vi "FGV_REWORK_DIAGNOSTICS_records_display.vi"(4 "front_panel_reference":refnum<vi>, 6 "SQL_listbox_reference":refnum<vi>, 7 "options":T2, 8 "error_in":errorcluster, 11 "input":variant) -> (0 "error_out":errorcluster, 1 "all_info":T1)   [LabVIEW 2019]
uses:
  FGV_REWORK_DIAGNOSTICS_records_display.ctl
  REWORK_DIAGNOSTICS_all_info.ctl
  ini/typedef/REWORK_all_config_info.ctl
  ini/typedef/REWORK_main_ini_file.ctl
  queues/typedef/REWORK_queue_refnums.ctl
  queues/typedef/REWORK_MAIN_queue_element.ctl
  MAIN/REWORK_MAIN_sequence_state.ctl
  queues/typedef/REWORK_SCANNER_queue_element.ctl
  SCANNER/REWORK_SCANNER_sequence_state.ctl
  _misc/PLC_connection_status.ctl
  connection_indicators/FGV_REWORK_connection_indicators.ctl
  _misc/AULocalize/SubVIs/Get Localized Phrase Compact Interface 1D.vi
  _misc/AULocalize/SubVIs/Get Localized Phrase Compact Interface 0D.vi
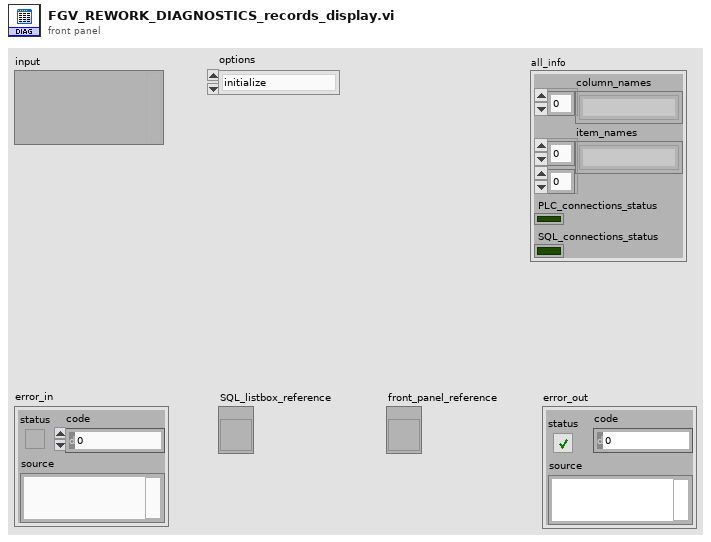
[diagram p1: front panel]
types:
  T1 = typedef "REWORK_DIAGNOSTICS_all_info.ctl" = cluster{"column_names":string[], "item_names":string[][], "PLC_connections_status":bool, "SQL_connections_status":bool}
  T2 = typedef "FGV_REWORK_DIAGNOSTICS_records_display.ctl" = enum16{"initialize", "set_PLC_IP", "set_PLC_Port", "set_PLC_connection_status", "set_SQL_connection_status", "get_all_info"}
  T3 = typedef "REWORK_all_config_info.ctl" = cluster{"main_ini_file":T4, "SQL Password":string, "queue_refnums":T5}
  T4 = typedef "REWORK_main_ini_file.ctl" = cluster{"SQL Driver":string, "SQL Server":string, "SQL Database":string, "SQL UID":string, "User table":string, "default language":string, "SCANNER COM port":u16, "SCANNER Baud rate":u32, "SCANNER Data bits":u16, "SCANNER Pairity":enum16{"None", "Odd", "Even", "Mark", "Space"}, "SCANNER Stop bits":u16, "SCANNER Flow control":u16, "SCANNER Termination char":u8, "ST 140 name":string, "ST 140 listener IP":string, "ST 140 listener port":u16, "logout timeout [ms]":i32}
  T5 = typedef "REWORK_queue_refnums.ctl" = cluster{"MAIN_queue":refnum<queue>, "SCANNER_queue":refnum<queue>, "SCANNER_data":refnum<queue>}
  T6 = typedef "FGV_REWORK_connection_indicators.ctl" = enum16{"initialize", "SQL_conn_ind_update", "PLC_conn_ind_update"}
  T7 = typedef "PLC_connection_status.ctl" = enum16{"Connected", "Waiting", "Error", "-"}
  T8 = cluster{"index (row)":i32, "disabled index (col)":i32}
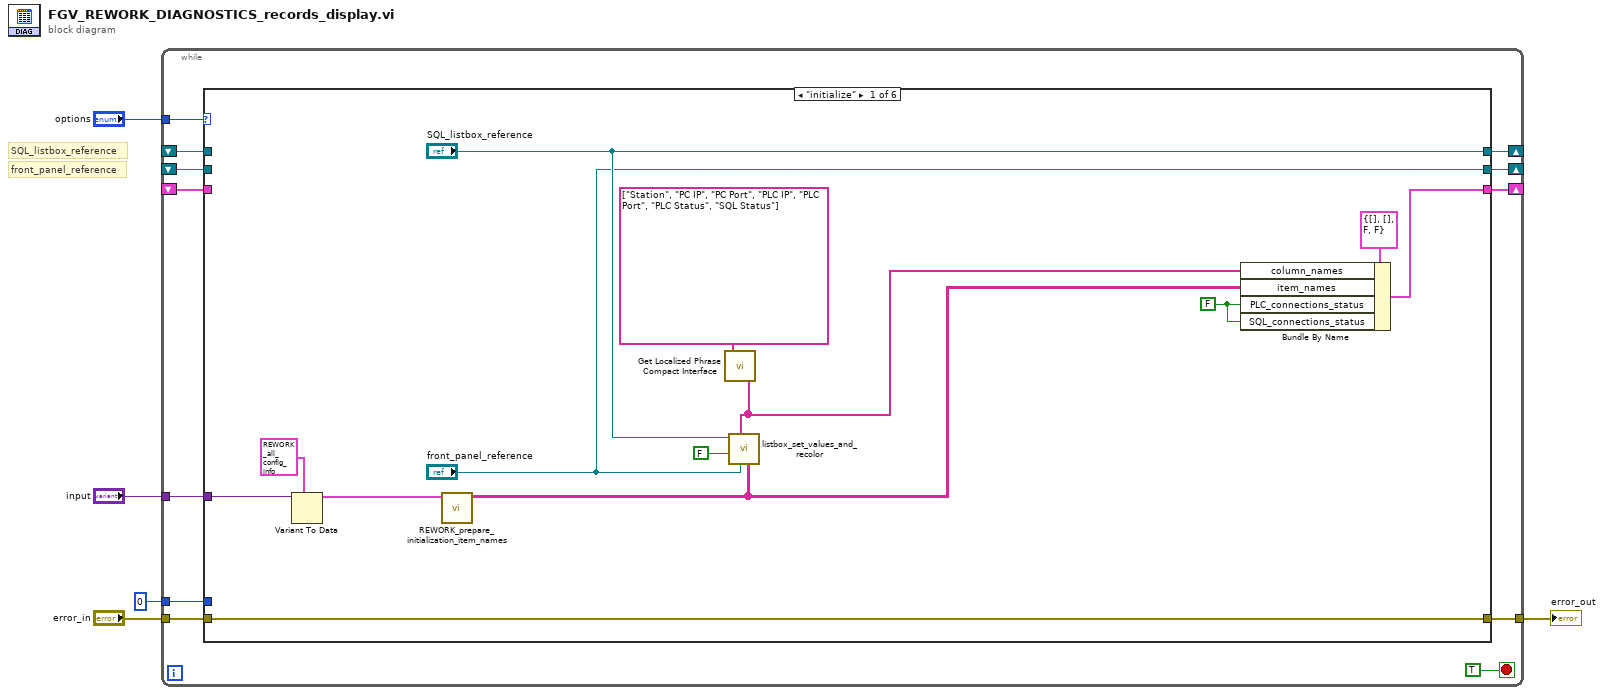
[diagram p0: block diagram]
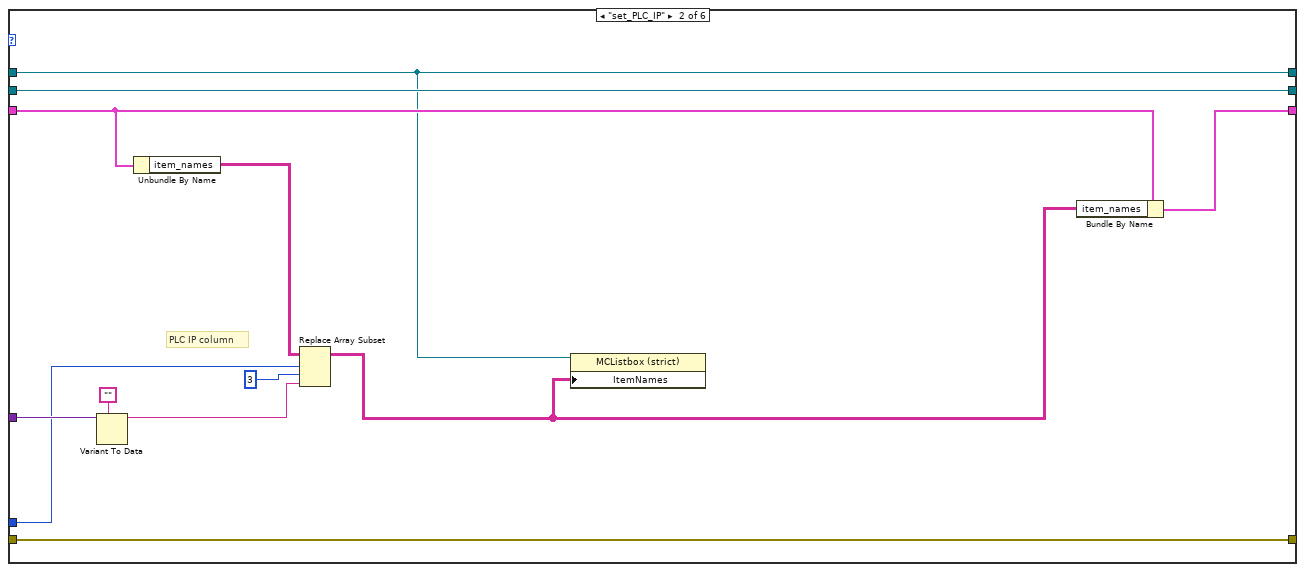
[diagram p2: hidden frame]
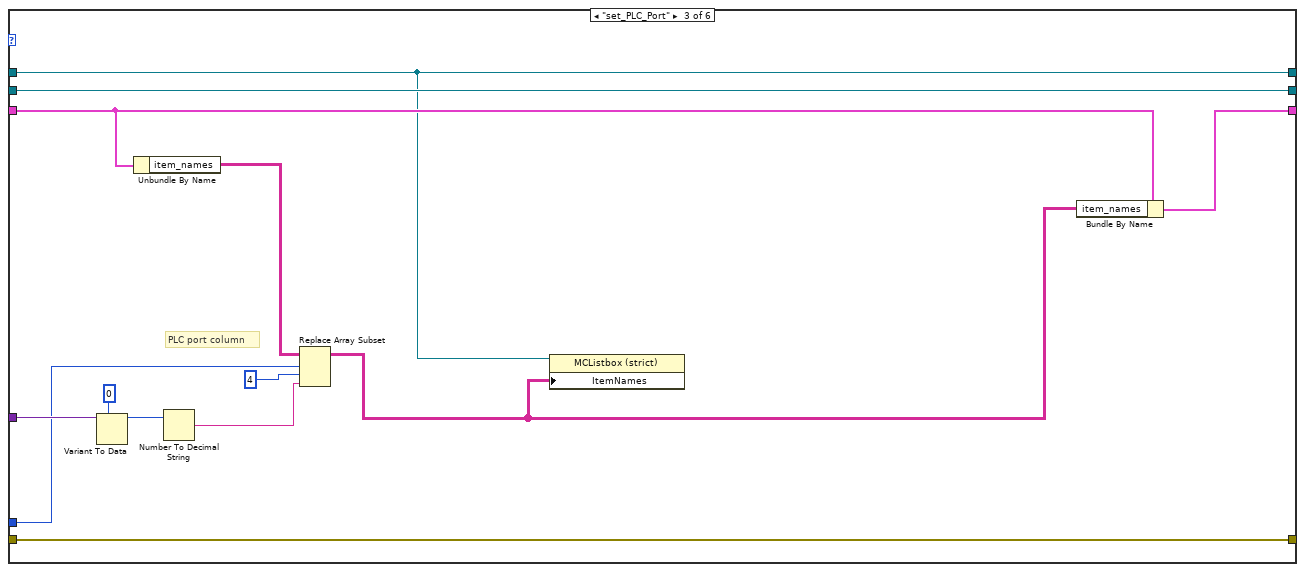
[diagram p3: hidden frame]
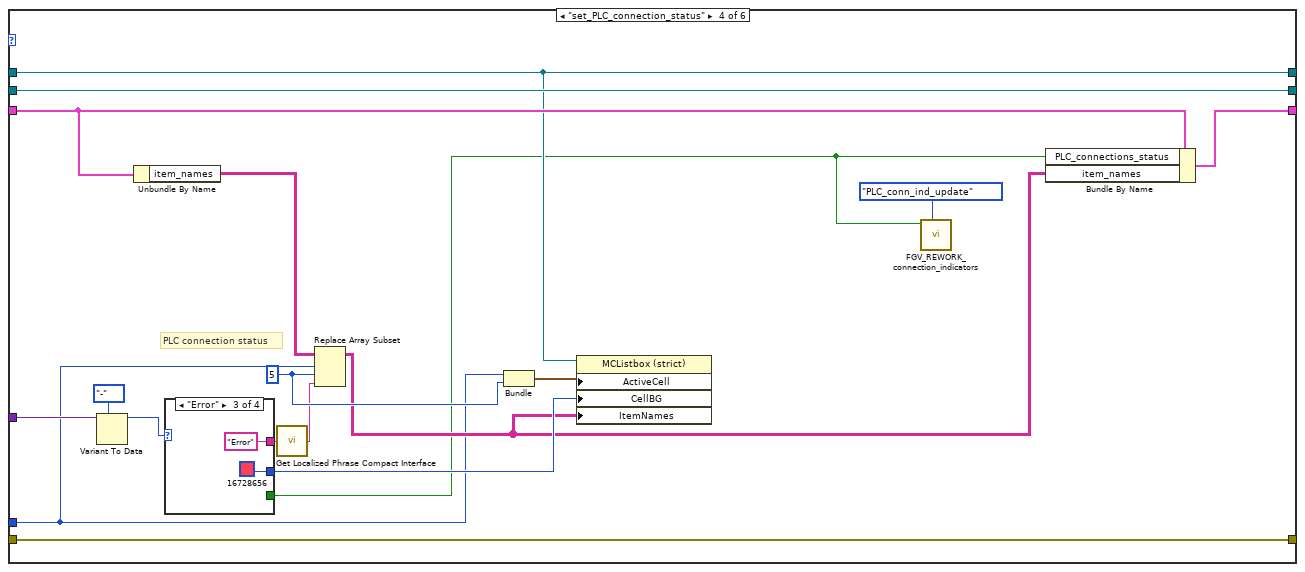
[diagram p4: hidden frame]
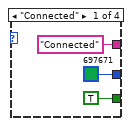
[diagram p5: hidden frame]
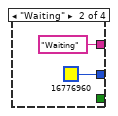
[diagram p6: hidden frame]
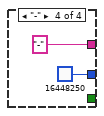
[diagram p7: hidden frame]
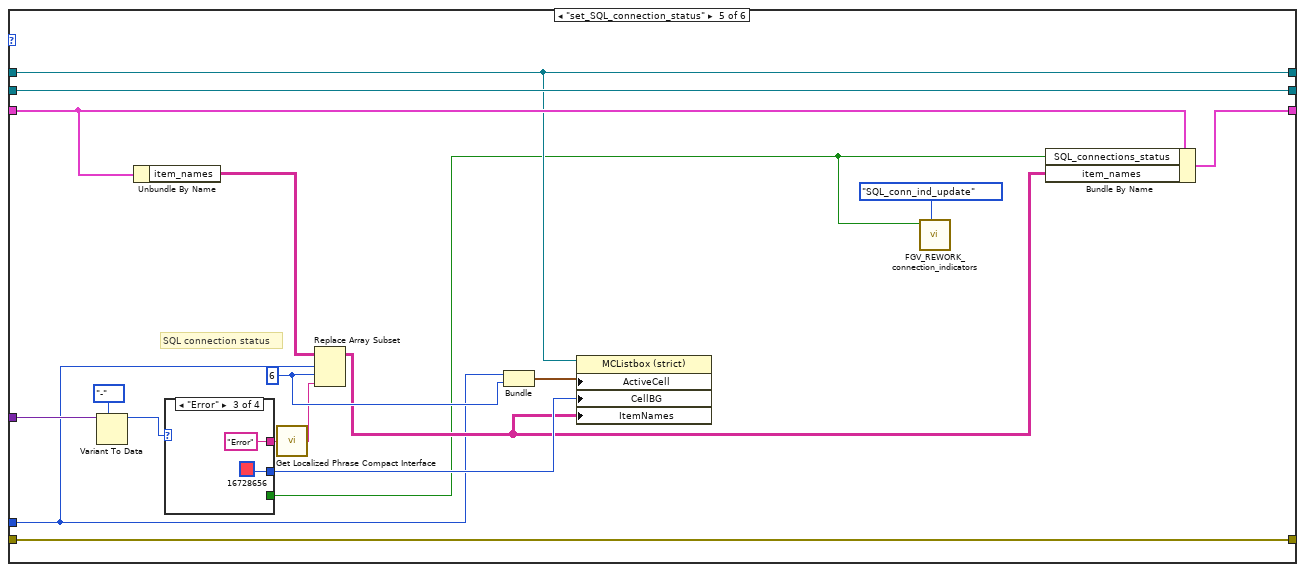
[diagram p8: hidden frame]
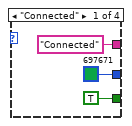
[diagram p9: hidden frame]
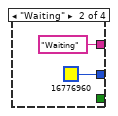
[diagram p10: hidden frame]
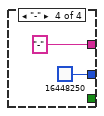
[diagram p11: hidden frame]
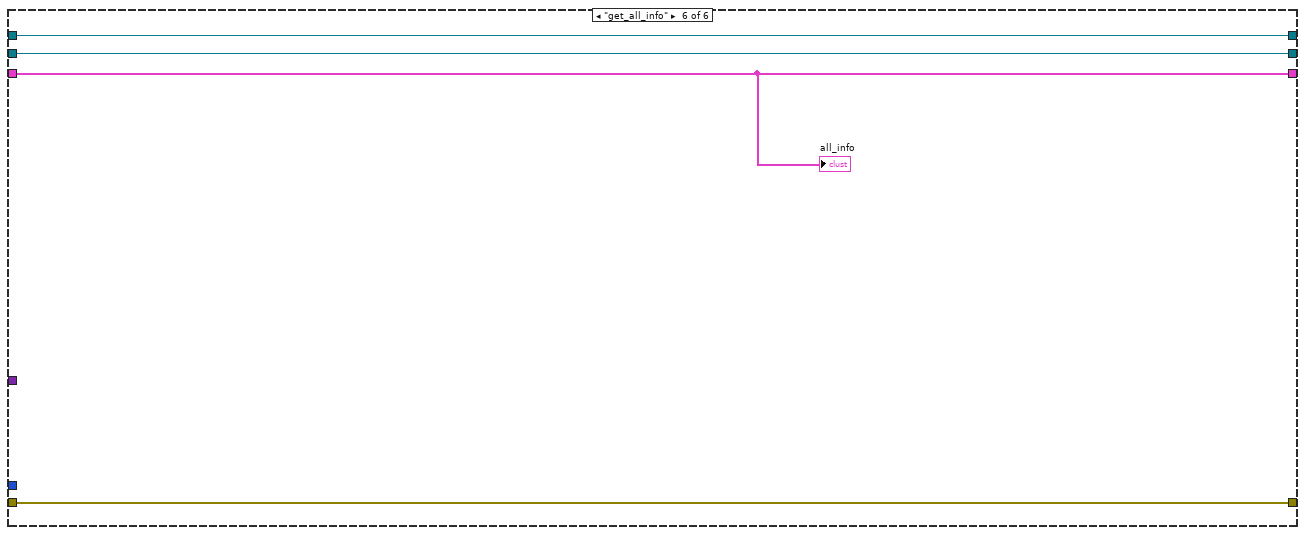
[diagram p12: hidden frame]
diagram:
  # "front_panel_reference"
  # "SQL_listbox_reference"
  n1 = while {
    tunnel: "options" -> [w16]
    tunnel: [w15] -> w5
    tunnel: "error_in" -> [w14]
    shift-right: [w13] -> _
    shift-left: _ -> [w12]
    shift-right: [w11] -> _
    shift-left: _ -> [w10]
    tunnel: "input" -> [w9]
    shift-right: [w8] -> _
    shift-left: _ -> [w7]
    tunnel: 0 ("index (row)") -> [w6]
    stop <- TRUE stop-if-true
    n2 = case shown="\"initialize\"" w16 {
      tunnel: [w30 w42 w55 w73 w100 w112] -> w15
      tunnel: w14 -> [w30 w42 w55 w73 w100 w112]
      tunnel: [w24 w40 w53 w71 w98 w113] -> w13
      tunnel: w12 -> [_ w39 w52 w70 w97 w113]
      tunnel: ["SQL_listbox_reference" w32 w44 w61 w88 w111] -> w11
      tunnel: w10 -> [_ w32 w44 w61 w88 w111]
      tunnel: w9 -> [w27 w41 w54 w72 w99 _]
      tunnel: ["front_panel_reference" w33 w45 w62 w89 w110] -> w8
      tunnel: w7 -> [_ w33 w45 w62 w89 w110]
      tunnel: w6 -> [_ w35 w50 w59 w86 _]
      frame "initialize" {
        w19 = FALSE ("PLC_connections_status")
        n3 = Variant To Data(type=T3 {"main_ini_file"={"SQL Driver"="", "SQL Server"="", "SQL Database"="", "SQL UID"="", "User table"="", "default language"="", "SCANNER COM port"=0, "SCANNER Baud rate"=0, "SCANNER Data bits"=0, "SCANNER Pairity"=enum."None", "SCANNER Stop bits"=10, "SCANNER Flow control"=0, "SCANNER Termination char"=0, "ST 140 name"="", "ST 140 listener IP"="", "ST 140 listener port"=0, "logout timeout [ms]"=0}, "SQL Password"="", "queue_refnums"={"MAIN_queue"=refnum, "SCANNER_queue"=refnum, "SCANNER_data"=refnum}} ("all_config_info"), Variant=w27) -> (data=w26:T3)  [unwired: 1 in, 1 out]
        n4 = call "REWORK_prepare_initialization_item_names.vi"("all_config_info"=w26) -> ("item_names"=w22:string[][])  [unwired: 10 in]
        n5 = call-poly "Get Localized Phrase Compact Interface.vi"("Key"=string[] ["Station", "PC IP", "PC Port", "PLC IP", "PLC Port", "PLC Status", "SQL Status"] ("column_names")) -> ("Translated Phrase"=w18:string[])
        n6 = call "listbox_set_values_and_recolor.vi"("item_names"=w22, "front_panel_reference"="front_panel_reference", "column_names"=w18, "Autosize? (T)"=FALSE, "multicolumn_listbox_reference_in"="SQL_listbox_reference") -> ()  [unwired: 5 in, 2 out]
        n7 = Bundle By Name(cluster=T1 {"column_names"=[], "item_names"=[], "PLC_connections_status"=FALSE, "SQL_connections_status"=FALSE} ("SQL_selection"), "column_names"=w18, "item_names"=w22, "PLC_connections_status"=w19, "SQL_connections_status"=w19) -> (w24:T1)
      }
      frame "set_PLC_IP" {
        # "PLC IP column"
        n8 = Variant To Data(type="", Variant=w41) -> (data=w36:string)  [unwired: 1 in, 1 out]
        n9 = Unbundle By Name(w39) -> ("item_names"=w37:string[][])
        n10 = Replace Array Subset(array=w37, new element=w36, index (row)=w35, index (col)=3 ("disabled index (col)")) -> (w31:string[][])
        n11 = property class="MCListbox (strict)"(reference=w32, "ItemNames"=w31) -> ()  [unwired: 1 in, 2 out]
        n12 = Bundle By Name(cluster=w39, "item_names"=w31) -> (w40:T1)
      }
      frame "set_PLC_Port" {
        # "PLC port column"
        n13 = Variant To Data(type=u16 0 ("remote port"), Variant=w54) -> (data=w47:u16)  [unwired: 1 in, 1 out]
        n14 = Unbundle By Name(w52) -> ("item_names"=w51:string[][])
        n15 = Number To Decimal String(number=w47) -> (decimal integer string=w46:string)  [unwired: 1 in]
        n16 = Replace Array Subset(array=w51, new element=w46, index (row)=w50, index (col)=4 ("disabled index (col)")) -> (w43:string[][])
        n17 = property class="MCListbox (strict)"(reference=w44, "ItemNames"=w43) -> ()  [unwired: 1 in, 2 out]
        n18 = Bundle By Name(cluster=w52, "item_names"=w43) -> (w53:T1)
      }
      frame "set_PLC_connection_status" {
        w63 = 5 ("disabled index (col)")
        # "PLC connection status"
        n19 = Variant To Data(type=PLC_connection_status."-", Variant=w72) -> (data=w67:T7)  [unwired: 1 in, 1 out]
        n20 = Unbundle By Name(w70) -> ("item_names"=w69:string[][])
        n21 = case shown="\"Error\"" w67 {
          tunnel: ["Connected" "Waiting" "Error" "-"] -> w66
          tunnel: [u32 697671 u32 16776960 u32 16728656 u32 16448250] -> w65
          tunnel: [TRUE _ _ _] -> w57
          frame "Connected" {
          }
          frame "Waiting" {
          }
          frame "Error" {
          }
          frame "-" {
          }
        }
        n22 = call-poly "Get Localized Phrase Compact Interface.vi"("Key"=w66) -> ("Translated Phrase"=w56:string)
        n23 = Replace Array Subset(array=w69, new element=w56, index (row)=w59, index (col)=w63) -> (w60:string[][])
        n24 = Bundle("index (row)"=w59, "disabled index (col)"=w63) -> (w64:T8)  [unwired: 1 in]
        n25 = property class="MCListbox (strict)"(reference=w61, "ActiveCell"=w64, "CellBG"=w65, "ItemNames"=w60) -> ()  [unwired: 1 in, 2 out]
        n26 = call "FGV_REWORK_connection_indicators.vi"("options"=FGV_REWORK_connection_indicators."PLC_conn_ind_update", "status"=w57) -> ()  [unwired: 9 in, 1 out]
        n27 = Bundle By Name(cluster=w70, "PLC_connections_status"=w57, "item_names"=w60) -> (w71:T1)
      }
      frame "set_SQL_connection_status" {
        w90 = 6 ("disabled index (col)")
        # "SQL connection status"
        n28 = Variant To Data(type=PLC_connection_status."-", Variant=w99) -> (data=w94:T7)  [unwired: 1 in, 1 out]
        n29 = Unbundle By Name(w97) -> ("item_names"=w96:string[][])
        n30 = case shown="\"Error\"" w94 {
          tunnel: ["Connected" "Waiting" "Error" "-"] -> w93
          tunnel: [u32 697671 u32 16776960 u32 16728656 u32 16448250] -> w92
          tunnel: [TRUE _ _ _] -> w84
          frame "Connected" {
          }
          frame "Waiting" {
          }
          frame "Error" {
          }
          frame "-" {
          }
        }
        n31 = call-poly "Get Localized Phrase Compact Interface.vi"("Key"=w93) -> ("Translated Phrase"=w83:string)
        n32 = Replace Array Subset(array=w96, new element=w83, index (row)=w86, index (col)=w90) -> (w87:string[][])
        n33 = Bundle("index (row)"=w86, "disabled index (col)"=w90) -> (w91:T8)  [unwired: 1 in]
        n34 = property class="MCListbox (strict)"(reference=w88, "ActiveCell"=w91, "CellBG"=w92, "ItemNames"=w87) -> ()  [unwired: 1 in, 2 out]
        n35 = call "FGV_REWORK_connection_indicators.vi"("options"=FGV_REWORK_connection_indicators."SQL_conn_ind_update", "status"=w84) -> ()  [unwired: 9 in, 1 out]
        n36 = Bundle By Name(cluster=w97, "SQL_connections_status"=w84, "item_names"=w87) -> (w98:T1)
      }
      frame "get_all_info" {
        "all_info" <- w113
      }
    }
  }
  "error_out" <- w5
